vi "Main_UI.vi"() -> ()   [LabVIEW 2023]
panel:
  out "Obtained_PSRR":dbl(graph) caption="Obtained PSRR"
  out "Error_Log_Table":string[][](table) caption="Error Log Table"
  in  "Error_Log":bool caption="Error Log"
  out "Last_Error_Details":T1 caption="Last Error Details"
  out "Last_Error_Details (dB)":dbl caption="Last Error Details (dB)"
  in  "Exit":bool
  in  "Wait_Time (sec)":dbl caption="Wait Time (sec)"
  out "Error?":bool
  # "PSRR Monitor"
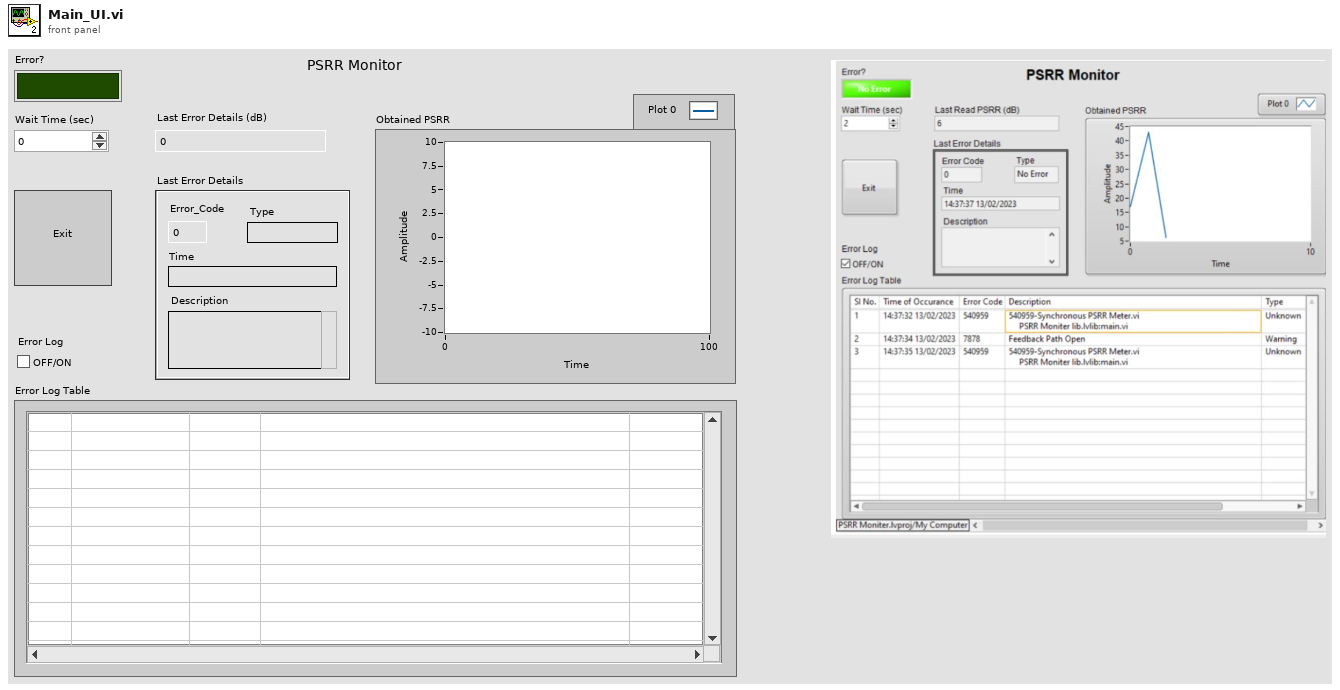
[diagram p1: front panel]
types:
  T1 = cluster{"Error_Code":dbl, "Type":string, "Time":string, "Description":string}
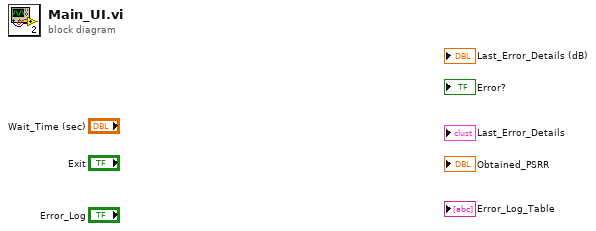
[diagram p0: block diagram]
diagram:
